vi "(SubVI) Trigger Options for DRT.vi"(4 "Enum":T1(ring)) -> (0 "trigger source array for DRT":i32[](array[numeric]), 1 "trigger option for DRT":i32)   [LabVIEW 2014]
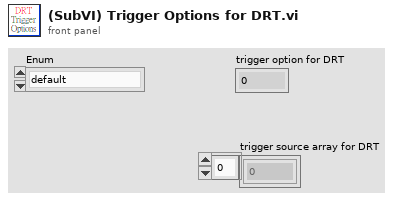
[diagram p1: front panel]
types:
  T1 = enum16{"default", "changing target position", "external trigger", "immediately"}
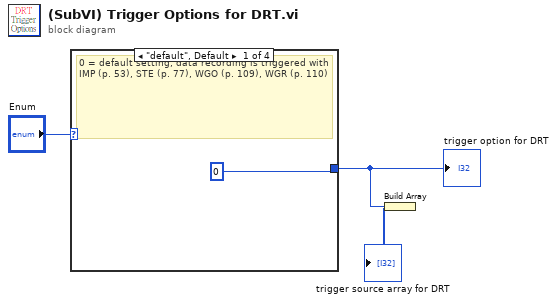
[diagram p0: block diagram]
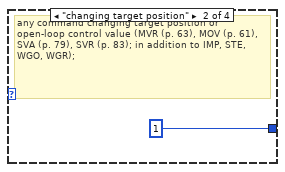
[diagram p2: hidden frame]
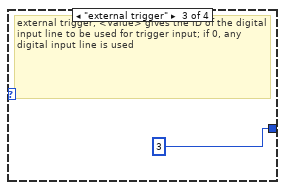
[diagram p3: hidden frame]
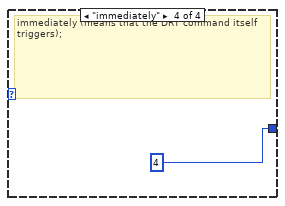
[diagram p4: hidden frame]
diagram:
  n1 = case shown="\"default\", Default" "Enum" {
    tunnel: [0 1 3 4] -> w2
    frame "default", Default {
      # "0 = default setting; data recording is triggered with \nIMP (p. 53), STE (p. 77), WGO (p. 109), WGR (p. 110)"
    }
    frame "changing target position" {
      # "any command changing target position or open-loop control value (MVR (p. 63), MOV (p. 61), SVA (p. 79), SVR (p. 83); in addition to IMP, STE, WGO, WGR);"
    }
    frame "external trigger" {
      # "external trigger; <Value> gives the ID of the digital input line to be used for trigger input; if 0, any digital input line is used"
    }
    frame "immediately" {
      # "immediately (means that the DRT command itself triggers);"
    }
  }
  "trigger option for DRT" <- w2
  n2 = Build Array(w2) -> (→"trigger source array for DRT":i32[])
